vi "JSON Object to Display Text.vi"(7 "Alphabetical Sort":bool, 10 "elements":string[](array[string]), 11 "Names":string[](array[string])) -> (3 "Display Text":string)   [LabVIEW 2019, in "JSONtext.lvlib"]
uses:
  JSONtext.lvlib
  JDP Science Common Utilities/JDP Utility.lvlib
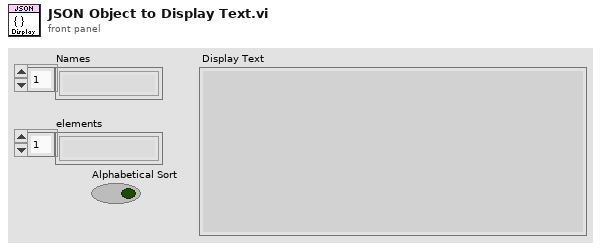
[diagram p1: front panel]
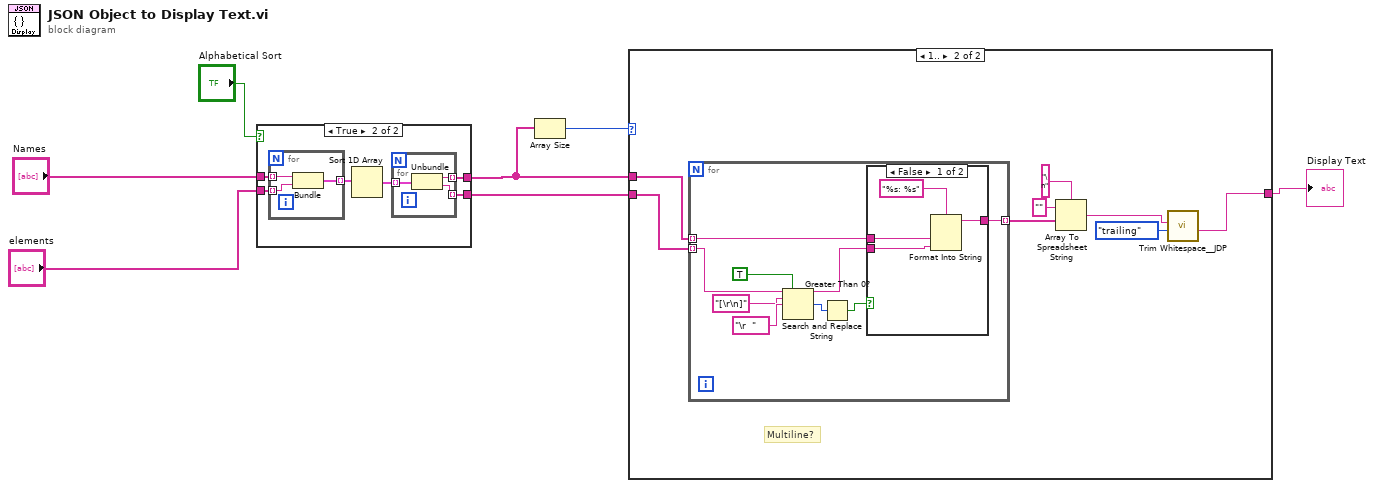
[diagram p0: block diagram]
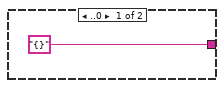
[diagram p2: hidden frame]
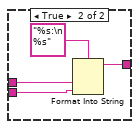
[diagram p3: hidden frame]
diagram:
  n1 = case shown="True" "Alphabetical Sort" {
    tunnel: "Names" -> [w9 w15]
    tunnel: "elements" -> [w8 w14]
    tunnel: [w9 w11] -> w4
    tunnel: [w8 w10] -> w3
    frame False {
    }
    frame True {
      n2 = for {
        tunnel: w15 -> [w21] mode=indexing
        tunnel: w14 -> [w20] mode=indexing
        tunnel: [w19] -> w13 mode=indexing
        n3 = Bundle(w21, "String"=w20) -> (w19:cluster{string, "String":string})  [unwired: 1 in]
      }
      n4 = Sort 1D Array(array=w13) -> (sorted array=w12:cluster{string, "String":string}[])
      n5 = for {
        tunnel: w12 -> [w18] mode=indexing
        tunnel: [w17] -> w10 mode=indexing
        tunnel: [w16] -> w11 mode=indexing
        n6 = Unbundle(w18) -> (w16:string, "String"=w17:string)
      }
    }
  }
  n7 = Array Size(array=w4) -> (size(s)=w5:i32)
  n8 = case shown="1.." w5 {
    tunnel: w4 -> [_ w30]
    tunnel: w3 -> [_ w29]
    tunnel: ["{}" w23] -> w2
    frame ..0 {
    }
    frame 1.. {
      # "Multiline?"
      n9 = for {
        tunnel: w30 -> [w39] mode=indexing
        tunnel: w29 -> [w34] mode=indexing
        tunnel: [w38] -> w28 mode=indexing
        n10 = Search and Replace String(replace all?=TRUE ("replace all? (F)"), input string=w34, search string="[\r\n]", replace string="\r  " ("search string")) -> (result string=w33:string, number of replacements=w31:i32)  [unwired: 4 in, 2 out]
        n11 = Greater Than 0?(x=w31) -> (x > 0?=w32:bool)
        n12 = case shown="False" w32 {
          tunnel: w39 -> [w42 w46]
          tunnel: [w41 w45] -> w38
          tunnel: w33 -> [w40 w44]
          frame False {
            n13 = Format Into String(format string="%s: %s", w42, w40) -> (resulting string=w41:string)  [unwired: 2 in, 1 out]
          }
          frame True {
            n14 = Format Into String(format string="%s:\n  %s", w46, w44) -> (resulting string=w45:string)  [unwired: 2 in, 1 out]
          }
        }
      }
      n15 = Array To Spreadsheet String(delimiter (Tab)="\n", array=w28, 3:"" ("format string")) -> (spreadsheet string=w25:string)
      n16 = call "Trim Whitespace__JDP.vi"("Remove (leading and trailing)"=enum16{"leading", "trailing", "both"}."trailing", "String in"=w25) -> ("String out"=w23:string)  [unwired: 5 in]
    }
  }
  "Display Text" <- w2
